vi "Load Calibration to TSM Site Data.vi"(0 "TSM context":T1, 5 "Cal File Path":path, 11 "error in":errorcluster) -> (15 "error out":errorcluster)   [LabVIEW 2020]
doc: "Loads calibration data obtained from the Acoustic Calibration File into TSM Site Data for each site."
uses:
  <vilib>/NI_TestStand_SemiconductorModule/NI_TestStand_Semiconductor_Module.lvlibp/PinMap/General/SemiconductorModuleContext.ctl
  398c8a69-9a96-41a5-b92f-a19b52f65231.vi
  <vilib>/NI_TestStand_SemiconductorModule/NI_TestStand_Semiconductor_Module.lvlibp
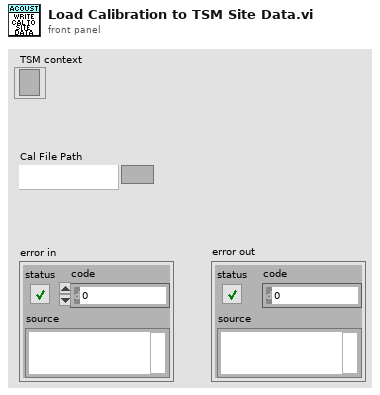
[diagram p1: front panel]
types:
  T1 = typedef "NI_TestStand_Semiconductor_Module.lvlibp/SemiconductorModuleContext.ctl" = refnum<k7>
  T2 = typedef "Acoustic Cal Data Cluster.ctl" = cluster{"Site Number":i32, "Serial Number":u32, "Ref Mic Sensitivity":dbl, "SPL Axis":dbl[], "Frequency Axis":dbl[], "Speaker Vp":dbl[][], "Ref Mic Cal File Data":string[][], "Speaker Vp Axis":dbl[], "SPL Measurements":dbl[][]}
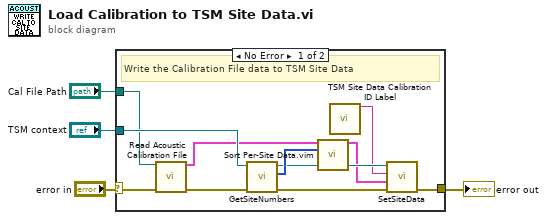
[diagram p0: block diagram]
diagram:
  n1 = case shown="No Error" "error in" {
    selector: "error in" -> [w13 w16]
    tunnel: [w15 w16] -> w4
    tunnel: "TSM context" -> [w14 _]
    tunnel: "Cal File Path" -> [w12 _]
    frame No Error {
      # "Write the Calibration File data to TSM Site Data"
      n2 = call "Read Acoustic Calibration File.vi"("Cal File Path"=w12, "error in (no error)"=w13) -> ("Per Site Acoustic Cal Data"=w9:T2[], "error out"=w11:errorcluster)  [unwired: 12 in]
      n3 = call <vilib>:"GetSiteNumbers.vi"("error in (no error)"=w11, "Semiconductor Module Context"=w14) -> ("error out"=w8:errorcluster, "Site Numbers"=w10:i32[], "Semiconductor Module Context Out"=w7:T1)  [unwired: 6 in, 1 out]
      n4 = call "Sort Per-Site Data.vim"("Per Site Unsorted Array In"=w9, "Site Numbers"=w10) -> ("Per Site Sorted Array Out"=w6:T2[])  [unwired: 13 in]
      n5 = call "TSM Site Data Calibration ID Label.vi"() -> ("Calibration Data Id"=w5:string)  [unwired: 15 in]
      n6 = call <vilib>:"SetSiteData.vi"("error in (no error)"=w8, "Site Data"=w6, "Data Id"=w5, "Semiconductor Module Context"=w7) -> ("error out"=w15:errorcluster)  [unwired: 5 in, 1 out]
    }
    frame Error {
      # "Error - Do Nothing"
    }
  }
  "error out" <- w4
